vi "MainTest.vi"() -> ()   [LabVIEW 2017]
uses:
  HITRAN-Line-Cluster.ctl
  D:/Data/SSoftware-VIs/labview-mongodb-csharp/C#/mongodb-dll/MongoLabVIEW/bin/Release/MongoLabVIEW.dll
  MongoLabVIEW/bin/Release/MongoLabVIEW.dll
panel:
  out "# lines":i32
  out "convertionTime (ms)":u32
  out "selectionTime (ms)":u32
  in  "limitInteger":i32=100
  in  "sortString":string="{param_intensity_weighted_abundace: -1}"
  in  "filterString":string="{ trans_nu: { $gte: 7246, $lte: 7352 }, trans_molec_id: 1 }"
  in  "selectionString":string="{ _id: false }"
  out "Lines":T1[](array[typedef])
  out "GetNumberOfDocs":i64
  in  "collectionName":string="hitran_2012"
  in  "databaseName":string="hitran"
  in  "connectionString":string="mongodb://tulpe:27017"
  # "MongoDB LabVIEW DLL Test"
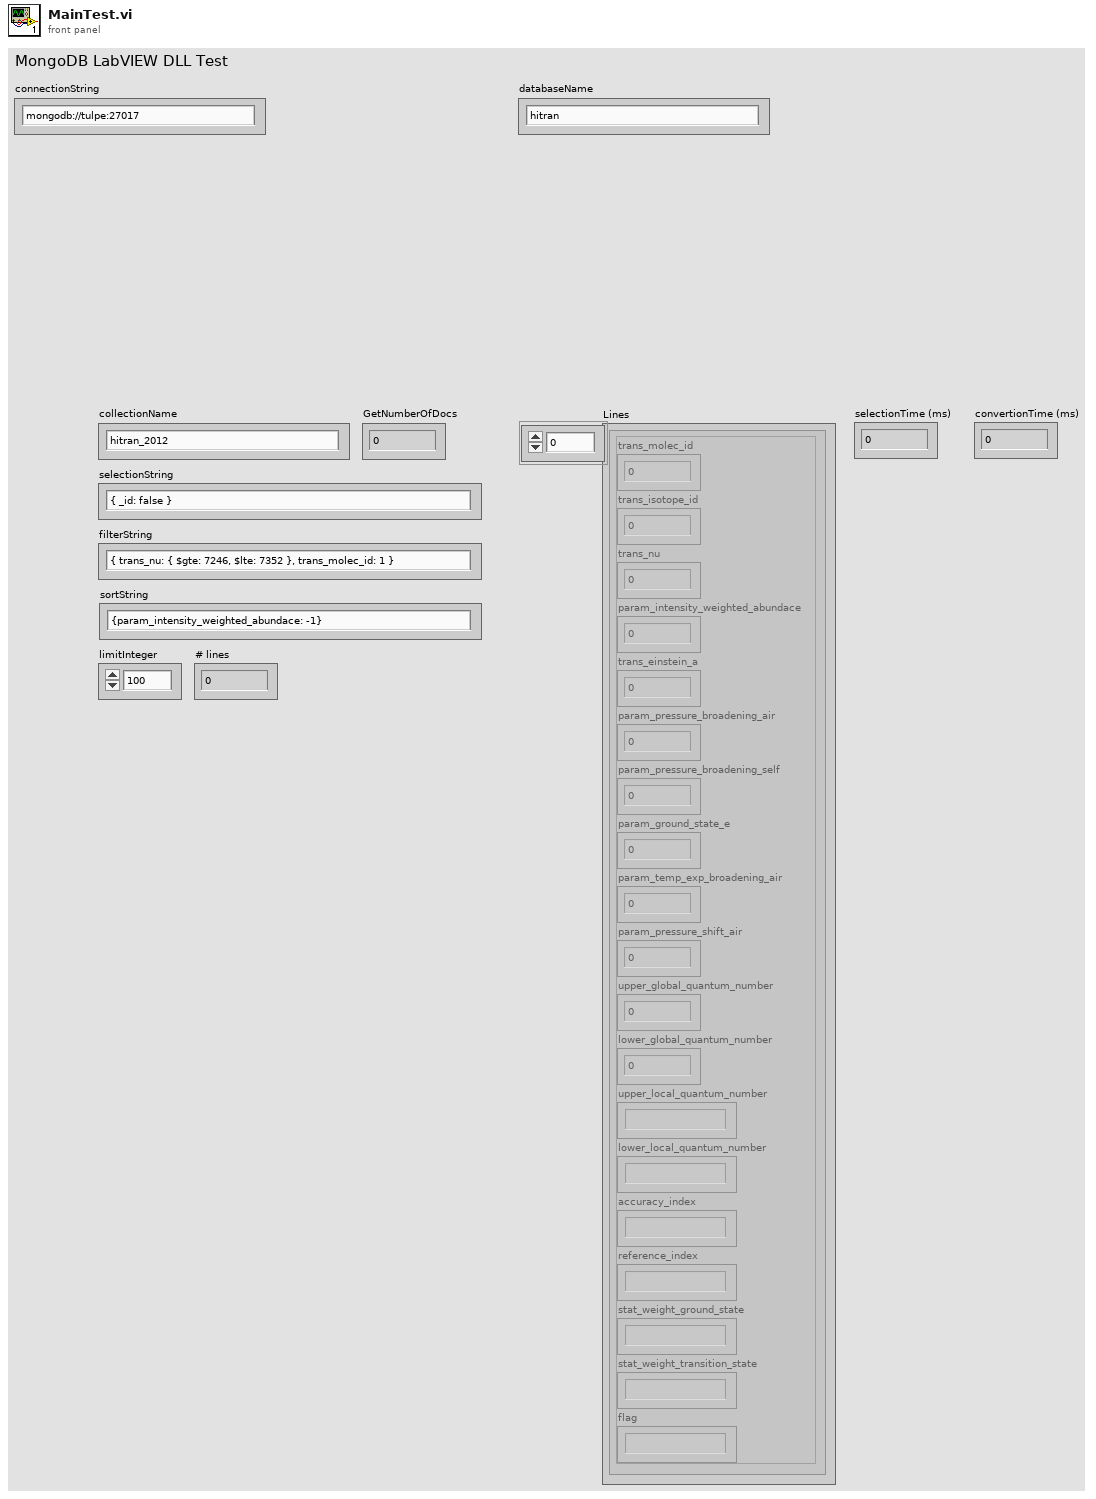
[diagram p1: front panel]
types:
  T1 = typedef "HITRAN-Line-Cluster.ctl" = cluster{"trans_molec_id":i32, "trans_isotope_id":i32, "trans_nu":dbl, "param_intensity_weighted_abundace":dbl, "trans_einstein_a":dbl, "param_pressure_broadening_air":dbl, "param_pressure_broadening_self":dbl, "param_ground_state_e":dbl, "param_temp_exp_broadening_air":dbl, "param_pressure_shift_air":dbl, "upper_global_quantum_number":i32, "lower_global_quantum_number":i32, "upper_local_quantum_number":string, "lower_local_quantum_number":string, "accuracy_index":string, "reference_index":string, "stat_weight_ground_state":string, "stat_weight_transition_state":string, "flag":string}
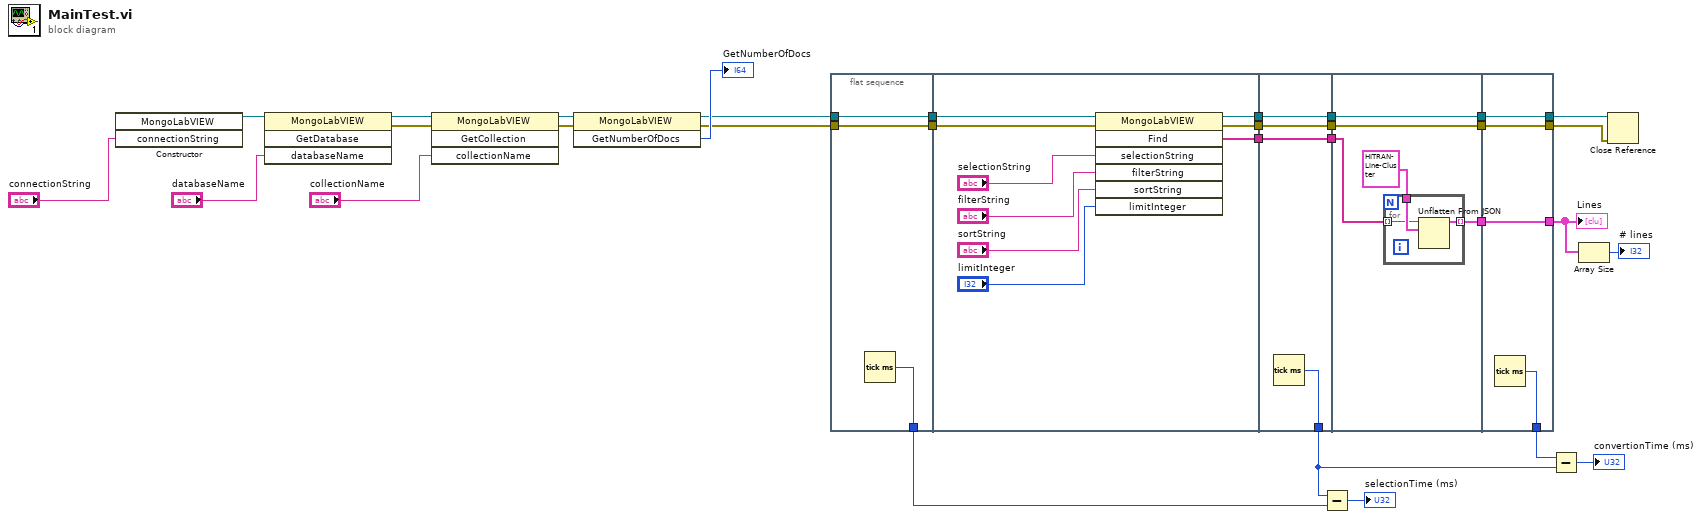
[diagram p0: block diagram]
diagram:
  n1 = constructor class="MongoLabVIEW"("connectionString"="connectionString") -> (reference out=w1:refnum<k24>)  [unwired: 3 in, 3 out]
  n2 = invoke class="MongoLabVIEW" method="GetDatabase"(reference=w1, "databaseName"="databaseName") -> (reference out=w29:refnum<k24>, error out=w28:errorcluster)  [unwired: 2 in, 2 out]
  n3 = invoke class="MongoLabVIEW" method="GetCollection"(reference=w29, error in=w28, "collectionName"="collectionName") -> (reference out=w26:refnum<k24>, error out=w25:errorcluster)  [unwired: 1 in, 2 out]
  n4 = invoke class="MongoLabVIEW" method="GetNumberOfDocs"(reference=w26, error in=w25) -> (reference out=w23:refnum<k24>, error out=w22:errorcluster, "GetNumberOfDocs"=→"GetNumberOfDocs":i64)  [unwired: 1 in]
  n5 = flat-sequence {
    tunnel: w22 -> [w33]
    tunnel: w23 -> [w34]
    tunnel: [w34] -> w19
    tunnel: [w33] -> w18
    tunnel: [w32] -> w8
    tunnel: w19 -> [w43]
    tunnel: w18 -> [w42]
    tunnel: [w41] -> w17
    tunnel: [w40] -> w16
    tunnel: [w35] -> w15
    tunnel: w17 -> [w47]
    tunnel: w16 -> [w46]
    tunnel: w15 -> [w45]
    tunnel: [w47] -> w14
    tunnel: [w46] -> w13
    tunnel: [w45] -> w12
    tunnel: [w44] -> w6
    tunnel: w14 -> [w52]
    tunnel: w13 -> [w51]
    tunnel: w12 -> [w49]
    tunnel: [w52] -> w11
    tunnel: [w51] -> w10
    tunnel: [w48] -> w9
    tunnel: [w57] -> w3
    tunnel: [w58] -> w20
    tunnel: [w59] -> w21
    tunnel: w11 -> [w59]
    tunnel: w10 -> [w58]
    tunnel: w9 -> [w57]
    tunnel: [w56] -> w7
    frame #0 {
      n6 = Tick Count (ms)() -> (millisecond timer value=w32:u32)
    }
    frame #1 {
      n7 = invoke class="MongoLabVIEW" method="Find"(reference=w43, error in=w42, "selectionString"="selectionString", "filterString"="filterString", "sortString"="sortString", "limitInteger"="limitInteger") -> (reference out=w41:refnum<k24>, error out=w40:errorcluster, "Find"=w35:string[])  [unwired: 1 in, 4 out]
    }
    frame #2 {
      n8 = Tick Count (ms)() -> (millisecond timer value=w44:u32)
    }
    frame #3 {
      n9 = for {
        tunnel: T1 {"trans_molec_id"=0, "trans_isotope_id"=0, "trans_nu"=0.0, "param_intensity_weighted_abundace"=0.0, "trans_einstein_a"=0.0, "param_pressure_broadening_air"=0.0, "param_pressure_broadening_self"=0.0, "param_ground_state_e"=0.0, "param_temp_exp_broadening_air"=0.0, "param_pressure_shift_air"=0.0, "upper_global_quantum_number"=0, "lower_global_quantum_number"=0, "upper_local_quantum_number"="", "lower_local_quantum_number"="", "accuracy_index"="", "reference_index"="", "stat_weight_ground_state"="", "stat_weight_transition_state"="", "flag"=""} ("HITRAN-Line-Cluster") -> [w55]
        tunnel: [w54] -> w48 mode=indexing
        tunnel: w49 -> [w53] mode=indexing
        n10 = Unflatten From JSON(JSON string=w53, type and defaults=w55) -> (value=w54:T1)  [unwired: 5 in, 1 out]
      }
    }
    frame #4 {
      n11 = Tick Count (ms)() -> (millisecond timer value=w56:u32)
    }
  }
  n12 = Subtract(x=w6, y=w8) -> (x-y=→"selectionTime (ms)":u32)
  n13 = Subtract(x=w7, y=w6) -> (x-y=→"convertionTime (ms)":u32)
  n14 = Array Size(array=w3) -> (size(s)=→"# lines":i32)
  n15 = Close Reference(reference=w21, error in (no error)=w20) -> ()  [unwired: 1 out]
  "Lines" <- w3
